vi "SIStringToNumeric.vi"(11 "SI number":string) -> (3 "Number":dbl, 5 "OK?":bool)   [LabVIEW 2020]
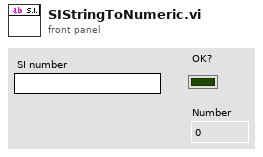
[diagram p1: front panel]
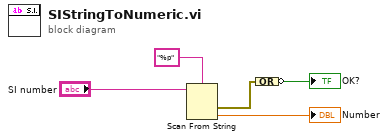
[diagram p0: block diagram]
diagram:
  n1 = Scan From String(format string="%p", input string="SI number") -> (error out=w4:errorcluster, output 1=→"Number":dbl)  [unwired: 3 in, 2 out]
  n2 = Compound Arithmetic op=OR(w4) -> (invert →"OK?":bool)
